vi "Get Request Type.vi"(8 "error in (no error)":errorcluster, 11 "GetSourceActive in":refnum<class "GetSourceActive.lvclass">) -> (0 "error out":errorcluster, 2 "Request Type":string, 3 "GetSourceActive out":refnum<class "GetSourceActive.lvclass">)   [LabVIEW 2020, in "obs-websocket.lvlib" / "GetSourceActive.lvclass"]
uses:
  GetSourceActive.lvclass
  GetSourceActive.lvclass/GetSourceActive.ctl
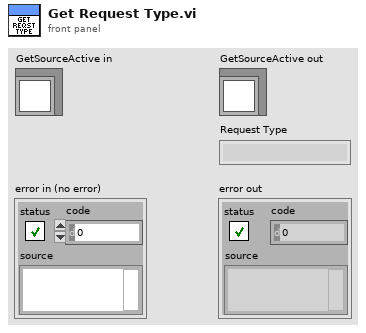
[diagram p1: front panel]
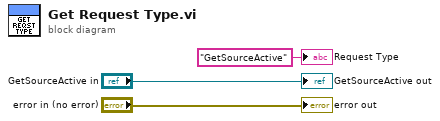
[diagram p0: block diagram]
diagram:
  "error out" <- "error in (no error)"
  "GetSourceActive out" <- "GetSourceActive in"
  "Request Type" <- "GetSourceActive" ("Request Type")
